vi "Filter Configuration Files.vi"(1 "Generated Files in":string[][](array[string])) -> (0 "Generated Files out":string[][](array[string]))   [LabVIEW 2018, in ".LVLIBP CD XML Updater.lvlib" / "Project XML Editor.lvclass"]
uses:
  Project XML Editor.lvclass
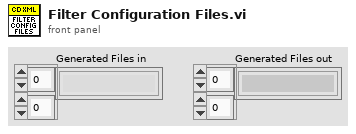
[diagram p1: front panel]
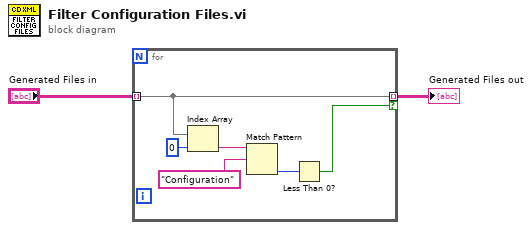
[diagram p0: block diagram]
diagram:
  n1 = for {
    tunnel: "Generated Files in" -> [w3] mode=indexing
    tunnel: [w3] -> w2 mode=indexing if=w4
    n2 = Index Array(array=w3, index=0) -> (element=w7:string)
    n3 = Match Pattern(string=w7, regular expression="Configuration") -> (offset past match=w5:i32)  [unwired: 1 in, 3 out]
    n4 = Less Than 0?(x=w5) -> (x < 0?=w4:bool)
  }
  "Generated Files out" <- w2
